vi "Init Msg Output.vi"() -> (3 "Stopped Msg Output out":refnum<class "--Stopped Msg Output.lvclass">)   [LabVIEW 2025, in "jettl.lvlib" / "Stopped jettl Msg.lvlib" / "--Stopped Msg Output.lvclass"]
uses:
  --Stopped Msg Output.lvclass
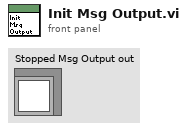
[diagram p1: front panel]
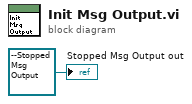
[diagram p0: block diagram]
diagram:
  "Stopped Msg Output out" <- refnum<class "--Stopped Msg Output.lvclass"> refnum ("Stopped Msg Output out")
